vi "AnyActive.vi"(8 "error in (no error)":errorcluster, 11 "S4GUI in":refnum<class "S4GUI.lvclass">) -> (0 "error out":errorcluster, 3 "S4GUI out":refnum<class "S4GUI.lvclass">)   [LabVIEW 2018, in "S4GUI.lvclass"]
uses:
  S4GUI.lvclass
  S4GUI.lvclass/S4GUI.ctl
  Acquisition/Acquisition.lvclass
  Channel/Channel.lvclass
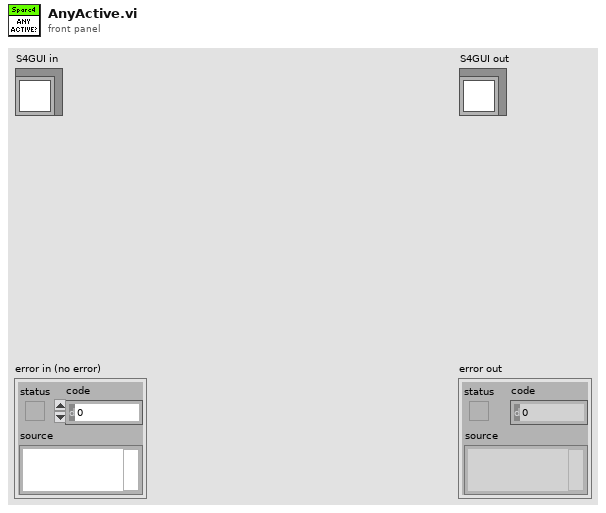
[diagram p1: front panel]
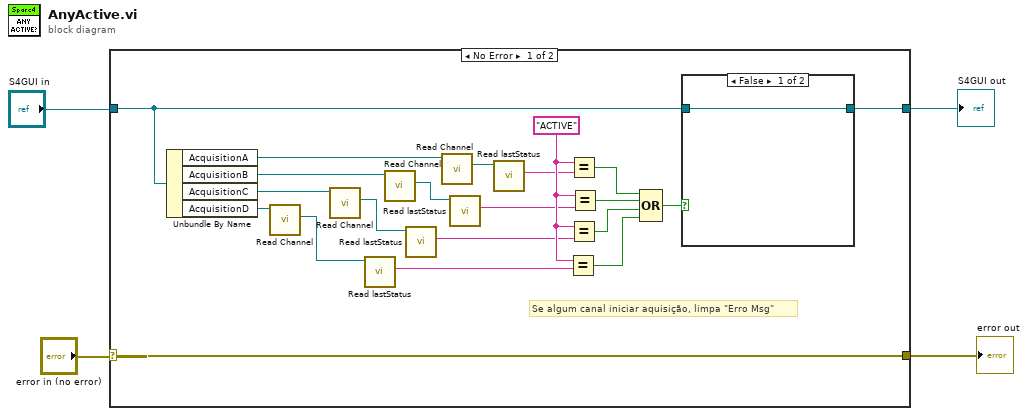
[diagram p0: block diagram]
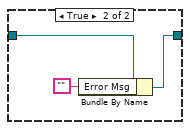
[diagram p2: hidden frame]
diagram:
  n1 = case shown="No Error" "error in (no error)" {
    selector: "error in (no error)" -> [w25 w31]
    tunnel: [w25 w31] -> w1
    tunnel: [w14 w30] -> w2
    tunnel: "S4GUI in" -> [w15 w30]
    frame No Error {
      w12 = "ACTIVE"
      # "Se algum canal iniciar aquisição, limpa \"Erro Msg\""
      n2 = Unbundle By Name(w15) -> ("AcquisitionA"=w24:refnum<class "Acquisition.lvclass">, "AcquisitionB"=w23:refnum<class "Acquisition.lvclass">, "AcquisitionC"=w22:refnum<class "Acquisition.lvclass">, "AcquisitionD"=w21:refnum<class "Acquisition.lvclass">)
      n3 = call-dynamic "Read Channel.vi"("Acquisition in"=w21) -> ("Channel.lvclass"=w6:refnum<class "Channel.lvclass">)  [unwired: 8 in, 2 out]
      n4 = call-dynamic "Read Channel.vi"("Acquisition in"=w22) -> ("Channel.lvclass"=w8:refnum<class "Channel.lvclass">)  [unwired: 8 in, 2 out]
      n5 = call-dynamic "Read lastStatus.vi"("Channel in"=w6) -> ("lastStatus"=w5:string)  [unwired: 8 in, 2 out]
      n6 = call-dynamic "Read Channel.vi"("Acquisition in"=w23) -> ("Channel.lvclass"=w10:refnum<class "Channel.lvclass">)  [unwired: 8 in, 2 out]
      n7 = call-dynamic "Read lastStatus.vi"("Channel in"=w8) -> ("lastStatus"=w7:string)  [unwired: 8 in, 2 out]
      n8 = call-dynamic "Read Channel.vi"("Acquisition in"=w24) -> ("Channel.lvclass"=w13:refnum<class "Channel.lvclass">)  [unwired: 8 in, 2 out]
      n9 = call-dynamic "Read lastStatus.vi"("Channel in"=w10) -> ("lastStatus"=w9:string)  [unwired: 8 in, 2 out]
      n10 = call-dynamic "Read lastStatus.vi"("Channel in"=w13) -> ("lastStatus"=w11:string)  [unwired: 8 in, 2 out]
      n11 = Equal?(x=w12, y=w5) -> (x = y?=w17:bool)
      n12 = Equal?(x=w12, y=w11) -> (x = y?=w20:bool)
      n13 = Equal?(x=w12, y=w7) -> (x = y?=w18:bool)
      n14 = Equal?(x=w12, y=w9) -> (x = y?=w19:bool)
      n15 = Compound Arithmetic op=OR(w20, w19, w18, w17) -> (w16:bool)
      n16 = case shown="False" w16 {
        tunnel: w15 -> [w26 w29]
        tunnel: [w26 w28] -> w14
        frame False {
        }
        frame True {
          n17 = Bundle By Name(cluster=w29, "Error Msg"="") -> (w28:refnum<class "S4GUI.lvclass">)
        }
      }
    }
    frame Error {
    }
  }
  "error out" <- w1
  "S4GUI out" <- w2
